vi "Turn Heater On.vi"() -> ()   [LabVIEW 2012]
uses:
  Heater State.ctl
  Traffic Light Simulator/Controls/Traffic Light States (with Walk and Exit State).ctl
panel:
  in  "Boolean Indicator":bool
  in  "Queue Ref in":refnum<queue>
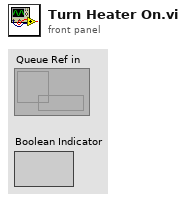
[diagram p1: front panel]
types:
  T1 = typedef "Heater State.ctl" = enum16{"Heater off", "Heating"}
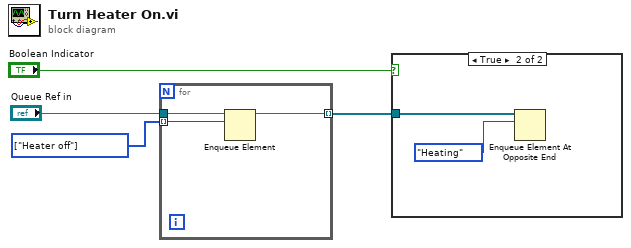
[diagram p0: block diagram]
diagram:
  w3 = T1[] [enum."Heater off"] items=["Heater off", "Heating"]
  n1 = for {
    tunnel: "Queue Ref in" -> [w7]
    tunnel: w3 -> [w6] mode=indexing
    tunnel: [w5] -> w1 mode=indexing
    n2 = Enqueue Element(queue=w7, element=w6) -> (queue out=w5:refnum<queue>)  [unwired: 2 in, 2 out]
  }
  n3 = case shown="True" "Boolean Indicator" {
    tunnel: w1 -> [_ w9]
    frame False {
    }
    frame True {
      n4 = Enqueue Element At Opposite End(queue=w9, element=Heater_State."Heating" ("Heater State")) -> ()  [unwired: 2 in, 3 out]
    }
  }
